vi "Call (async) JSON.vi"(4 "ArgumentsKw":string, 6 "Arguments":string, 7 "Options":string, 8 "error in (no error)":errorcluster, 9 "Notify result":bool, 10 "Topic URI":string, 11 "WAMP Client in":refnum<class "WAMP Client.lvclass">) -> (0 "error out":errorcluster, 2 "Call result notifier":refnum<notifier>, 3 "WAMP Client out":refnum<class "WAMP Client.lvclass">)   [LabVIEW 2020, in "wamplv.lvlib" / "WAMP Client.lvclass"]
uses:
  WAMP Client.lvclass
  TypeDefs/RESULT payload (JSON).ctl
  TypeDefs/Combined error.ctl
  TypeDefs/WAMP error.ctl
  WAMP Client.lvclass/WAMP Client.ctl
  Private/TypeDef/CALL request (JSON).ctl
  Private/TypeDef/Internal Message Type.ctl
  44dd0fb6-e4b1-424e-8704-d5c62803e1d5.vi
  <vilib>/Utility/error.llb/Error Cluster From Error Code.vi
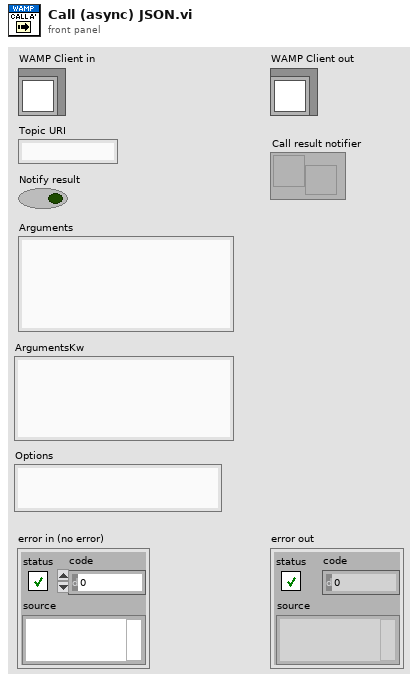
[diagram p1: front panel]
types:
  T1 = typedef "wamplv.lvlib/WAMP Client.lvclass/RESULT payload (JSON).ctl" = cluster{"Arguments Payload":string, "ArgumentKw Payload":string, "Topic":string, "Combined Error":T2}
  T2 = typedef "wamplv.lvlib/WAMP Client.lvclass/Combined error.ctl" = cluster{"Error?":bool, "WAMP Error":T3, "Error":errorcluster}
  T3 = typedef "wamplv.lvlib/WAMP Client.lvclass/WAMP error.ctl" = cluster{"Details":string, "ArgumentKw Payload":string, "Error?":bool, "Error URI":string, "Arguments Payload":string}
  T4 = typedef "wamplv.lvlib/WAMP Client.lvclass/CALL request (JSON).ctl" = cluster{"Topic URI":string, "Arguments":string, "ArgumentsKw":string, "Options":string, "Call result":refnum<notifier>}
  T5 = typedef "wamplv.lvlib/WAMP Client.lvclass/Internal Message Type.ctl" = enum16{"Subscribe", "Handle Subscribed", "Handle Event", "Unsubscribe", "Handle Unsubscribed", "Publish", "Handled Published", "Goodbye", "Handle Goodbye", "Call", "Handle Result", "Register", "Handle Registered", "Unregister", "Handle Unregistered", "Handle Invocation", "Yield", "Error"}
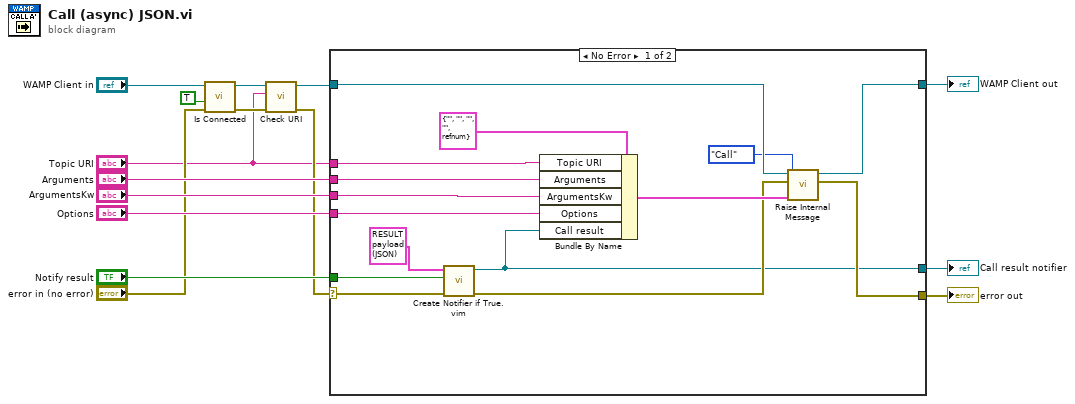
[diagram p0: block diagram]
diagram:
  n1 = call "Is Connected.vi"("error in"="error in (no error)", "Raise error if not connected"=TRUE, "WAMP Client in"="WAMP Client in") -> ("error out"=w6:errorcluster, "WAMP Client out"=w3:refnum<class "WAMP Client.lvclass">)  [unwired: 6 in, 1 out]
  n2 = call "Check URI.vi"("error in (no error)"=w6, "URI"="Topic URI", "WAMP Client in"=w3) -> ("error out"=w5:errorcluster, "WAMP Client out"=w1:refnum<class "WAMP Client.lvclass">)  [unwired: 5 in, 2 out]
  n3 = case shown="No Error" w5 {
    selector: w5 -> [w20 w32]
    tunnel: [w27 w32] -> w15
    tunnel: [w29 w31] -> w14
    tunnel: w1 -> [w30 w31]
    tunnel: "Topic URI" -> [w25 _]
    tunnel: "Arguments" -> [w24 _]
    tunnel: "ArgumentsKw" -> [w22 _]
    tunnel: "Options" -> [w21 _]
    tunnel: [w17 _] -> w10
    tunnel: "Notify result" -> [w18 _]
    frame No Error {
      n4 = call "Create Notifier if True.vim"("error in (no error)"=w20, "Boolean"=w18, "RESULT Payload"=T1 {"Arguments Payload"="", "ArgumentKw Payload"="", "Topic"="", "Combined Error"={"Error?"=FALSE, "WAMP Error"={"Details"="{}", "ArgumentKw Payload"="{}", "Error?"=FALSE, "Error URI"="", "Arguments Payload"=""}, "Error"={"status"=FALSE, "code"=0, "source"=""}}}) -> ("error out"=w19:errorcluster, "Notifier out"=w17:refnum<notifier>)  [unwired: 7 in]
      n5 = Bundle By Name(cluster=T4 {"Topic URI"="", "Arguments"="", "ArgumentsKw"="", "Options"="", "Call result"=refnum} ("Call Request"), "Topic URI"=w25, "Arguments"=w24, "ArgumentsKw"=w22, "Options"=w21, "Call result"=w17) -> (w23:T4)
      n6 = call "Raise Internal Message.vi"("Variant"=w23, "Internal Message Type"=Internal_Message_Type."Call", "error in (no error)"=w19, "WAMP Client in"=w30) -> ("error out"=w27:errorcluster, "WAMP Client out"=w29:refnum<class "WAMP Client.lvclass">)  [unwired: 6 in]
    }
    frame Error {
    }
  }
  "error out" <- w15
  "WAMP Client out" <- w14
  "Call result notifier" <- w10
